vi "Write Data.vi"(8 "error in (no error)":errorcluster, 9 "Name":string, 10 "Data":refnum<class "AbstractData.lvclass">, 11 "Observable Actor in":refnum<class "Observable Actor.lvclass">) -> (0 "error out":errorcluster, 3 "Observable Actor out":refnum<class "Observable Actor.lvclass">)   [LabVIEW 2014, in "Observable Actor.lvlib" / "Observable Actor.lvclass"]
uses:
  Observable Actor.lvclass
  Model/Data/AbstractData/AbstractData.lvclass
  Observable Actor.lvclass/Observable Actor.ctl
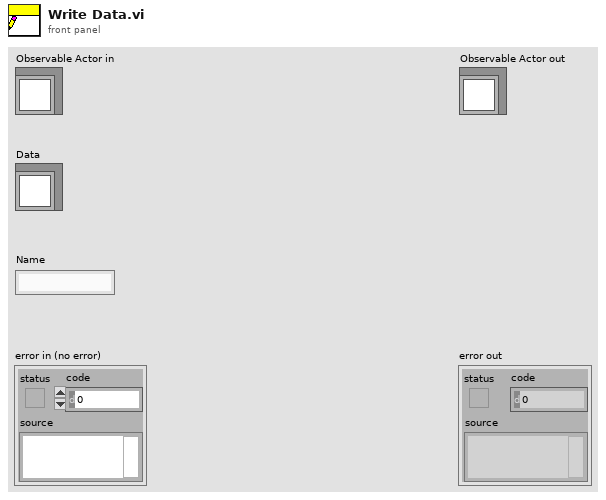
[diagram p1: front panel]
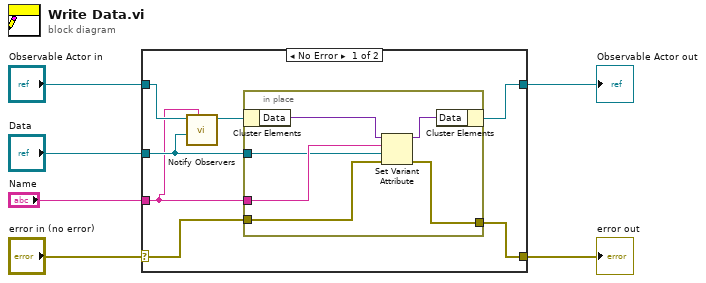
[diagram p0: block diagram]
diagram:
  n1 = case shown="No Error" "error in (no error)" {
    selector: "error in (no error)" -> [w7 w20]
    tunnel: [w13 w20] -> w5
    tunnel: [w12 w21] -> w2
    tunnel: "Observable Actor in" -> [w11 w21]
    tunnel: "Data" -> [w9 _]
    tunnel: "Name" -> [w8 _]
    frame No Error {
      n2 = call "Notify Observers.vi"("name"=w8, "value"=w9, "Observable Actor in"=w11) -> ("Observable Actor out"=w10:refnum<class "Observable Actor.lvclass">)  [unwired: 7 in, 1 out]
      n3 = in-place {
        in-place-border: w8 -> [w18]
        in-place-border: w9 -> [w17]
        in-place-border: w7 -> [w16]
        in-place-border: [w15] -> w13
        n4 = in-place-cluster #1(w10) -> ("Data"=w14:variant)
        n5 = Set Variant Attribute(Variant=w14, name=w18, value=w17, error in=w16) -> (Variant out=w19:variant, error out=w15:errorcluster)  [unwired: 1 out]
        n6 = in-place-cluster #1("Data"=w19) -> (w12:refnum<class "Observable Actor.lvclass">)
      }
    }
    frame Error {
    }
  }
  "error out" <- w5
  "Observable Actor out" <- w2
